vi "Execute.vi"(8 "error in (no error)":errorcluster, 9 "Workspace":T1, 10 "Control In":T2, 11 "Secure Syringe in":refnum<class "SecureRelease Syringe.lvclass">) -> (0 "error out":errorcluster, 2 "Control Out":T2, 3 "Secure Syringe out":refnum<class "SecureRelease Syringe.lvclass">)   [LabVIEW 2020, in "SecureRelease Syringe.lvclass"]
uses:
  SecureRelease Syringe.lvclass
  Controller/Controllers.ctl
  Controller/I-O/I-O.lvclass
  Controller/Dispenser/Dispenser.lvclass
  C:/Program Files (x86)/Aerotech/A3200/LabVIEW/2010/Bin/Aerotech.A3200.dll
  Program Files (x86)/Aerotech/A3200/LabVIEW/2010/Bin/Aerotech.A3200.dll
  Workspace/Workspace.ctl
  SecureRelease Syringe.lvclass/SecureRelease Syringe.ctl
  Controller/Motion/Motion.lvclass
  Dispense/Dispense.lvclass
  Controller/Motion/A3200/A3200.lvclass
  Controller/Controller.lvclass
  Workspace/Fixture.lvclass
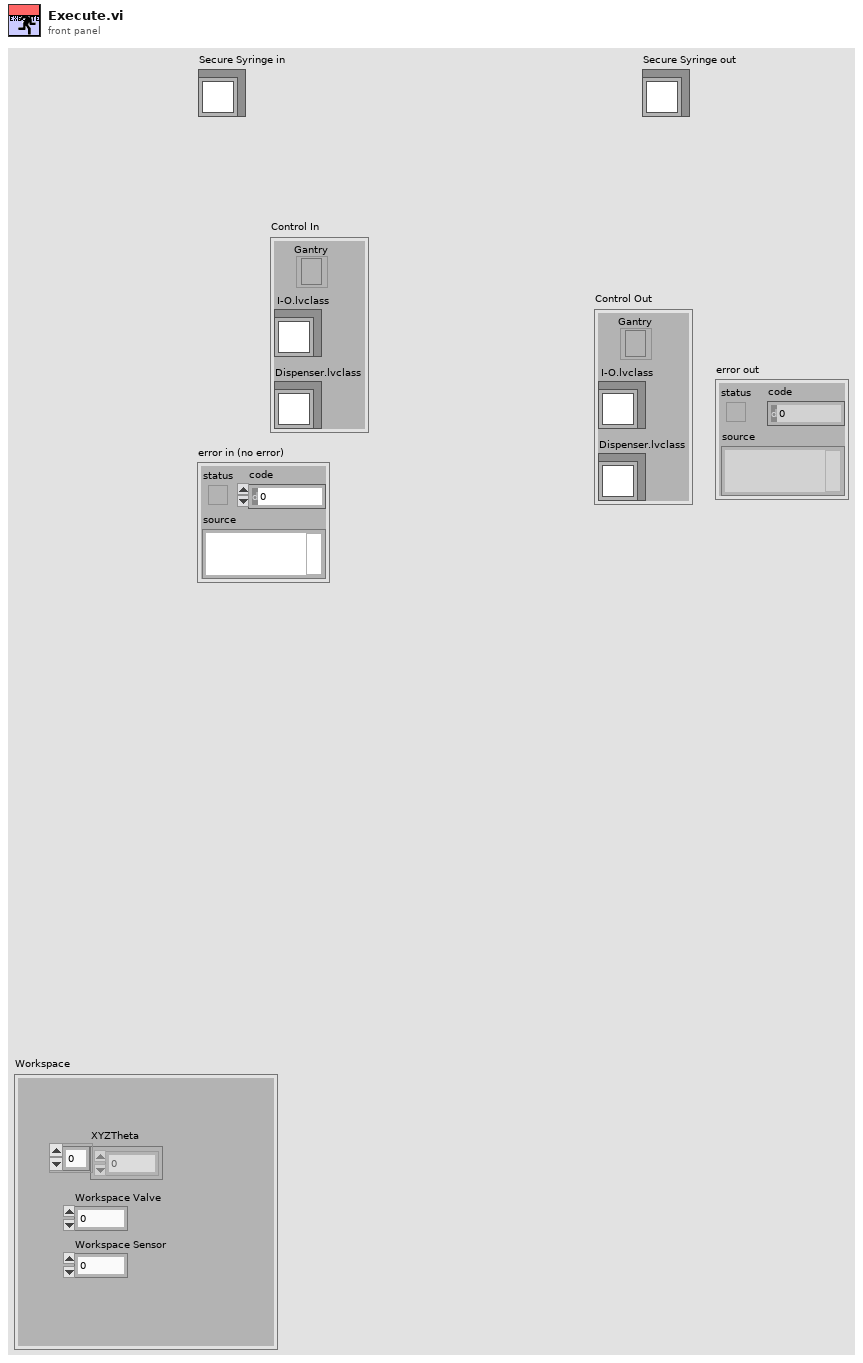
[diagram p1: front panel]
types:
  T1 = typedef "Fixture.lvclass/Workspace.ctl" = cluster{"XYZTheta":dbl[], "Workspace Valve":i32, "Workspace Sensor":i32}
  T2 = typedef "Controller.lvclass/Controllers.ctl" = cluster{"I-O.lvclass":refnum<class "I-O.lvclass">, "Dispenser.lvclass":refnum<class "Dispenser.lvclass">, "Gantry":refnum<k24>}
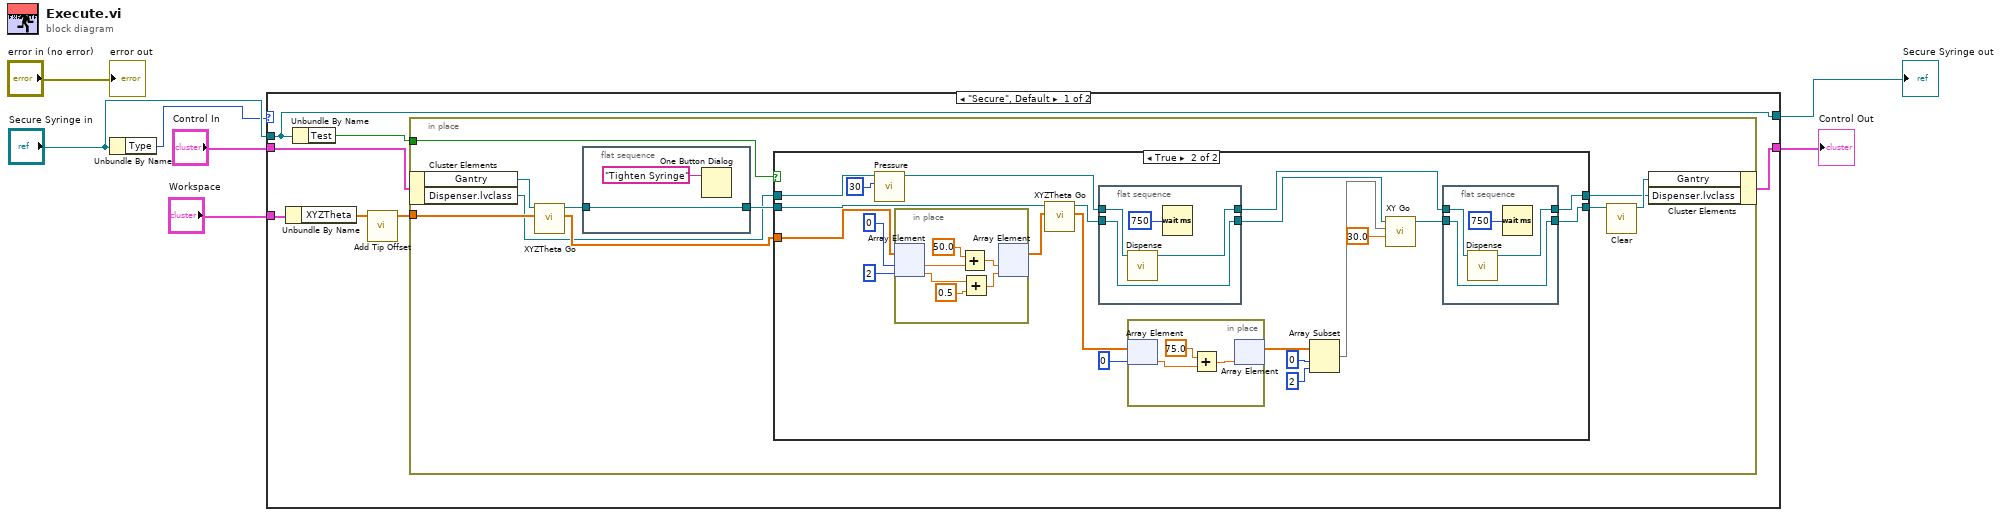
[diagram p0: block diagram]
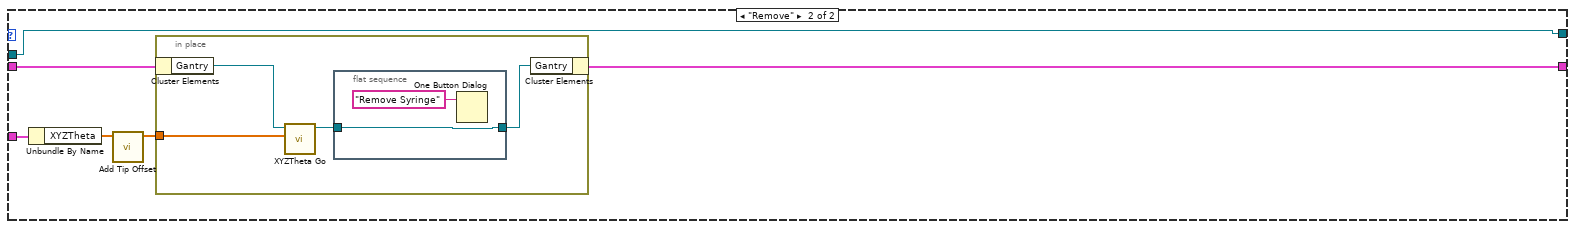
[diagram p3: hidden frame]
diagram:
  n1 = Unbundle By Name("Secure Syringe in") -> ("Type"=w1:enum16{"Secure", "Remove"})
  n2 = case shown="\"Secure\", Default" w1 {
    tunnel: "Workspace" -> [w14 w69]
    tunnel: "Secure Syringe in" -> [w10 w70]
    tunnel: [w10 w70] -> w5
    tunnel: "Control In" -> [w13 w71]
    tunnel: [w12 w72] -> w3
    frame "Secure", Default {
      n3 = Unbundle By Name(w14) -> ("XYZTheta"=w9:dbl[])
      n4 = Unbundle By Name(w10) -> ("Test"=w11:bool)
      n5 = call "Add Tip Offset.vi"("XYZTheta"=w9) -> ("XYZTheta"=w8:dbl[])  [unwired: 10 in]
      n6 = in-place {
        in-place-border: w8 -> [w23]
        in-place-border: w11 -> [w17]
        n7 = in-place-cluster #1(w13) -> ("Gantry"=w24:refnum<k24>, "Dispenser.lvclass"=w16:refnum<class "Dispenser.lvclass">)
        n8 = call "XYZTheta Go.vi"("XYZTheta In"=w23, "Gantry 2"=w24) -> ("XYZTheta Out"=w18:dbl[], "Gantry 3"=w22:refnum<k24>)  [unwired: 7 in, 1 out]
        n9 = flat-sequence {
          tunnel: [w65] -> w20
          tunnel: w22 -> [w65]
          frame #0 {
            n10 = One Button Dialog(message="Tighten Syringe") -> ()  [unwired: 1 in, 1 out]
          }
        }
        n11 = case shown="True" w17 {
          tunnel: w20 -> [w26 w47]
          tunnel: [w26 w36] -> w19
          tunnel: w18 -> [_ w46]
          tunnel: w16 -> [w25 w40]
          tunnel: [w25 w34] -> w15
          frame False {
          }
          frame True {
            n12 = call-dynamic "Pressure.vi"("Pressure"=i16 30, "Dispenser in"=w40) -> ("Dispenser out"=w37:refnum<class "Dispenser.lvclass">)  [unwired: 8 in, 1 out]
            n13 = in-place {
              n14 = in-place-array #2(w46, 0, 2) -> (w64:dbl, w62:dbl)
              n15 = Add(x=50.0, y=w64) -> (x+y=w59:dbl)
              n16 = Add(x=w62, y=0.5) -> (x+y=w60:dbl)
              n17 = in-place-array #2(w59, w60) -> (w43:dbl[])  [unwired: 2 out]
            }
            n18 = call "XYZTheta Go.vi"("XYZTheta In"=w43, "Gantry 2"=w47) -> ("XYZTheta Out"=w42:dbl[], "Gantry 3"=w38:refnum<k24>)  [unwired: 7 in, 1 out]
            n19 = flat-sequence {
              tunnel: [w55] -> w28
              tunnel: w38 -> [w55]
              tunnel: w37 -> [w54]
              tunnel: [w52] -> w35
              frame #0 {
                n20 = call-dynamic "Dispense.vi"("Dispenser in"=w54) -> ("Dispenser out"=w52:refnum<class "Dispenser.lvclass">)  [unwired: 9 in, 1 out]
                n21 = Wait (ms)(milliseconds to wait=u32 750) -> ()  [unwired: 1 out]
              }
            }
            n22 = in-place {
              n23 = in-place-array #3(w42, 0) -> (w58:dbl)
              n24 = Add(x=75.0, y=w58) -> (x+y=w56:dbl)
              n25 = in-place-array #3(w56) -> (w33:dbl[])  [unwired: 1 out]
            }
            n26 = Array Subset(array=w33, index=0, length=2) -> (w30:dbl[])
            n27 = call "XY Go.vi"("Speed"=30.0, "XY"=w30, "Gantry 2"=w28) -> ("Gantry 3"=w27:refnum<k24>)  [unwired: 7 in, 1 out]
            n28 = flat-sequence {
              tunnel: [w51] -> w36
              tunnel: w27 -> [w51]
              tunnel: w35 -> [w50]
              tunnel: [w48] -> w34
              frame #0 {
                n29 = call-dynamic "Dispense.vi"("Dispenser in"=w50) -> ("Dispenser out"=w48:refnum<class "Dispenser.lvclass">)  [unwired: 9 in, 1 out]
                n30 = Wait (ms)(milliseconds to wait=u32 750) -> ()  [unwired: 1 out]
              }
            }
          }
        }
        n31 = call "Clear.vi"("Gantry 2"=w19) -> ("Gantry 3"=w21:refnum<k24>)  [unwired: 9 in, 1 out]
        n32 = in-place-cluster #1("Gantry"=w21, "Dispenser.lvclass"=w15) -> (w12:T2)
      }
    }
    frame "Remove" {
      n33 = Unbundle By Name(w69) -> ("XYZTheta"=w68:dbl[])
      n34 = call "Add Tip Offset.vi"("XYZTheta"=w68) -> ("XYZTheta"=w67:dbl[])  [unwired: 10 in]
      n35 = in-place {
        in-place-border: w67 -> [w73]
        n36 = in-place-cluster #4(w71) -> ("Gantry"=w76:refnum<k24>)
        n37 = call "XYZTheta Go.vi"("XYZTheta In"=w73, "Gantry 2"=w76) -> ("Gantry 3"=w75:refnum<k24>)  [unwired: 7 in, 2 out]
        n38 = flat-sequence {
          tunnel: w75 -> [w78]
          tunnel: [w78] -> w74
          frame #0 {
            n39 = One Button Dialog(message="Remove Syringe") -> ()  [unwired: 1 in, 1 out]
          }
        }
        n40 = in-place-cluster #4("Gantry"=w74) -> (w72:T2)
      }
    }
  }
  "Secure Syringe out" <- w5
  "Control Out" <- w3
  "error out" <- "error in (no error)"
